vi "Kelvinox_Set_Monitor_Values.vi"(5 "System Monitor Variables (in)":T1) -> (1 "System Monitor Variables (out)":T1)   [LabVIEW 2019]
uses:
  Global/Global Variables/System Monitor Cluster.ctl
  Global/Global Variables/Data_Display_global.vi
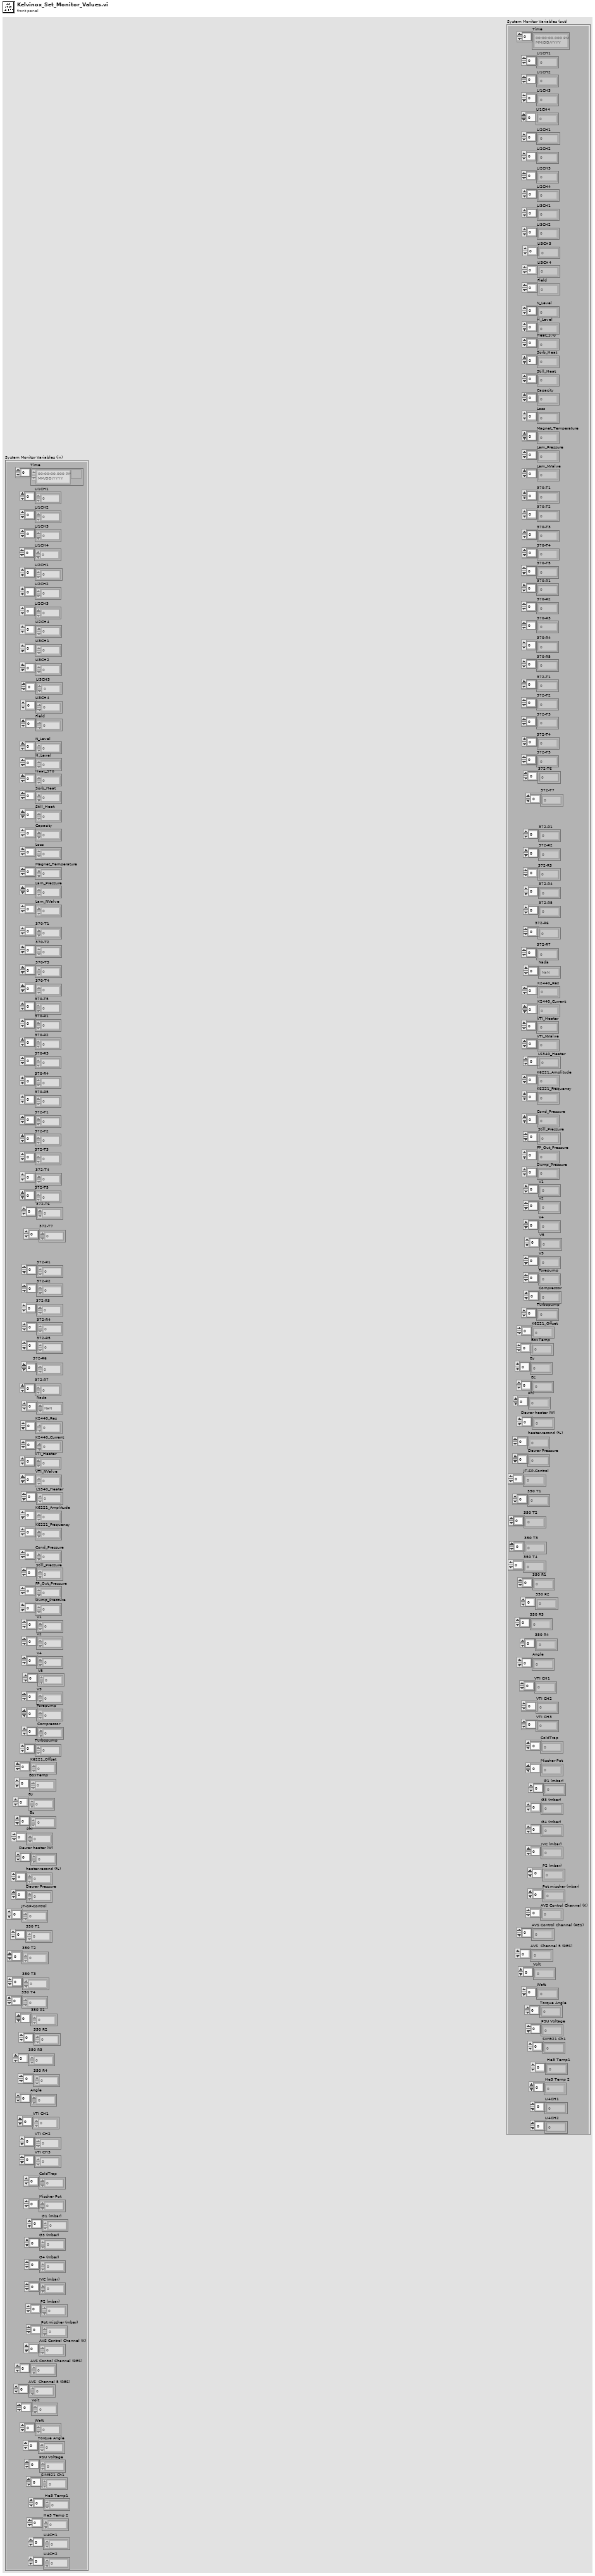
[diagram p1: front panel]
types:
  T1 = typedef "System Monitor Cluster.ctl" = cluster{"Time":timestamp[], "LI1CH1":dbl[], "LI1CH2":dbl[], "LI2CH1":dbl[], "LI2CH2":dbl[], "LI3CH1":dbl[], "LI3CH2":dbl[], "Field":dbl[], "N_Level":dbl[], "H_Level":dbl[], "Heat_370":dbl[], "Sorb_Heat":dbl[], "Still_Heat":dbl[], "Capacity":dbl[], "Loss":dbl[], "Magnet_Temperature":dbl[], "Lam_Pressure":dbl[], "Lam_NValve":dbl[], "370-T1":dbl[], "370-T2":dbl[], "370-T3":dbl[], "370-T4":dbl[], "370-T5":dbl[], "370-R1":dbl[], "370-R2":dbl[], "370-R3":dbl[], "370-R4":dbl[], "370-R5":dbl[], "372-T1":dbl[], "372-T2":dbl[], "372-T3":dbl[], "372-T4":dbl[], "372-T5":dbl[], "372-T6":dbl[], "372-R1":dbl[], "372-R2":dbl[], "372-R3":dbl[], "372-R4":dbl[], "372-R5":dbl[], "372-R6":dbl[], "Nada":dbl[], "K2440_Res":dbl[], "K2440_Current":dbl[], "VTI_Heater":dbl[], "VTI_NValve":dbl[], "LS340_Heater":dbl[], "K6221_Amplitude":dbl[], "K6221_Frequency":dbl[], "Cond_Pressure":dbl[], "Still_Pressure":dbl[], "FP_Out_Pressure":dbl[], "Dump_Pressure":dbl[], "V1":dbl[], "V2":dbl[], "V4":dbl[], "V5":dbl[], "V9":dbl[], "Forepump":dbl[], "Compressor":dbl[], "K6221_Offset":dbl[], "BoxTemp":dbl[], "By":dbl[], "Bz":dbl[], "Phi":dbl[], "heater-recond (%)":dbl[], "Dewar Pressure ":dbl[], "JT-SP-Control":dbl[], "350 T1":dbl[], "350 T2":dbl[], "350 T3":dbl[], "350 T4":dbl[], "350 R1":dbl[], "350 R2":dbl[], "350 R3":dbl[], "350 R4":dbl[], "Angle":dbl[], "VTI CH1":dbl[], "VTI CH2":dbl[], "VTI CH3":dbl[], "ColdTrap":dbl[], "Mischer Pot":dbl[], "G1 (mbar)":dbl[], "G3 (mbar) ":dbl[], "G4 (mbar)":dbl[], "IVC (mbar)":dbl[], "P2 (mbar) ":dbl[], "Pot mischer (mbar)":dbl[], "AVS Control Channel (K)":dbl[], "AVS Control Channel (RES)":dbl[], "AVS  Channel 5 (RES) ":dbl[], "LI3CH3":dbl[], "LI3CH4":dbl[], "LI1CH3":dbl[], "LI1CH4":dbl[], "LI2CH3":dbl[], "LI2CH4":dbl[], "Volt":dbl[], "Watt":dbl[], "Torque Angle":dbl[], "Dewar heater (W)":dbl[], "PSU Voltage":dbl[], "Turbopump":dbl[], "372-R7":dbl[], "372-T7":dbl[], "SIM921 Ch1":dbl[], " He3 Temp1":dbl[], " He3 Temp 2":dbl[], "LI4CH1":dbl[], "LI4CH2":dbl[]}
  T2 = typedef "Kelvinox_Status.ctl" = cluster{"V1":bool, "V2":bool, "Dump":u16, "V4":bool, "V5":bool, "V9":bool, "P1":dbl, "P2":dbl, "P3":dbl, "P4":dbl, "P5":dbl, "Turbo":bool, "Forepump":bool, "speed":dbl, "Sorb":dbl, "1K Pot":dbl, "Still":dbl, "Cold\nPlate":dbl, "MC":dbl, "4K":dbl, "Sample":dbl, "T-Setpoint":dbl, "MC Heater":dbl, "Still Heater":dbl, "Sorb Heater":dbl, "T Control active":bool, "Sorb Res":dbl, "1K Pot Res":dbl, "Still Res":dbl, "Cold Plate Res":dbl, "MC Res":dbl, "4K Res":dbl, "Sample Res":dbl, "Ramping":bool}
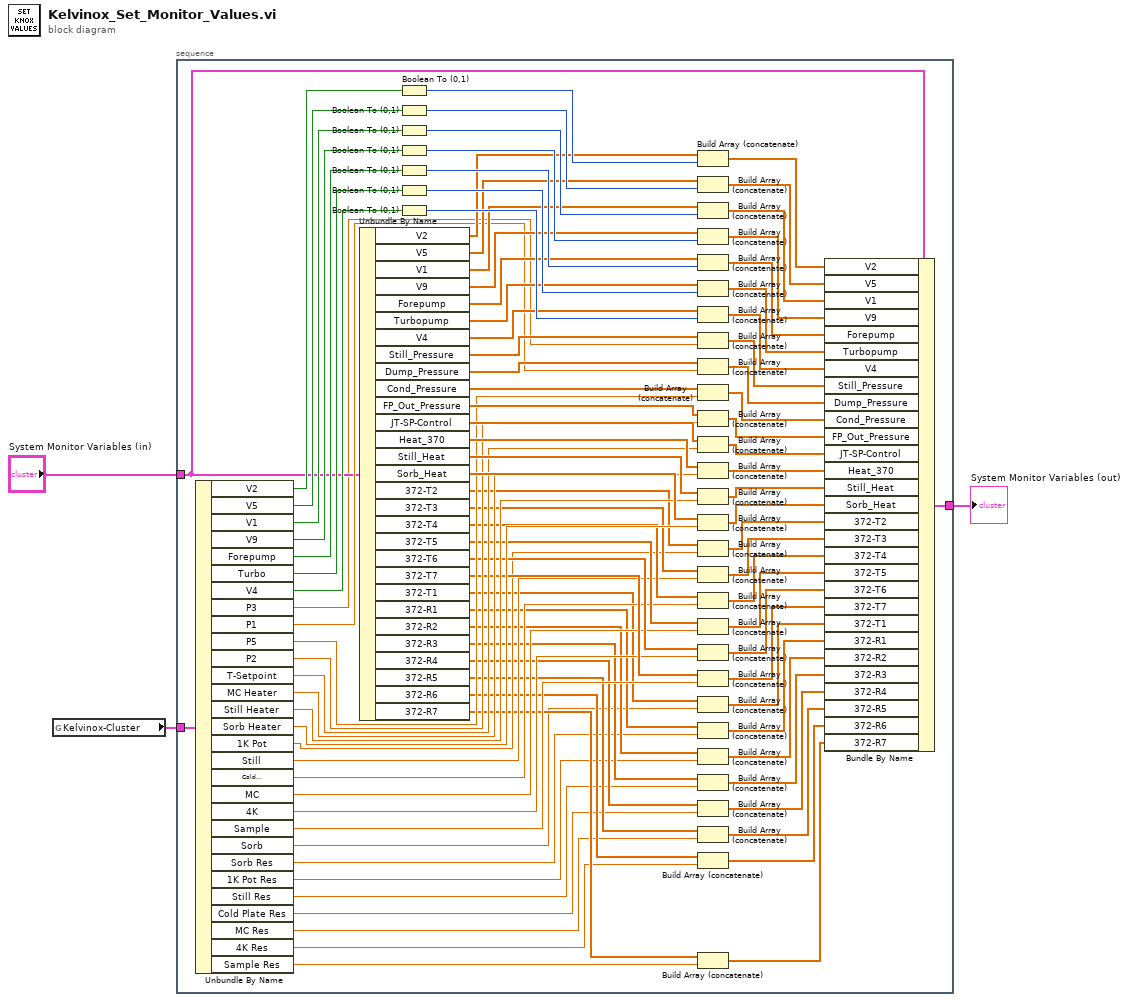
[diagram p0: block diagram]
diagram:
  n1 = global read "Data_Display_global.vi" "Kelvinox-Cluster"() -> (w1:T2)
  n2 = stacked-sequence {
    tunnel: "System Monitor Variables (in)" -> [w51]
    tunnel: [w62] -> w2
    tunnel: w1 -> [w100]
    frame #0 {
      n3 = Unbundle By Name(w100) -> ("V2"=w61:bool, "V5"=w60:bool, "V1"=w59:bool, "V9"=w58:bool, "Forepump"=w57:bool, "Turbo"=w56:bool, "V4"=w55:bool, "P3"=w50:dbl, "P1"=w52:dbl, "P5"=w54:dbl, "P2"=w53:dbl, "T-Setpoint"=w49:dbl, "MC Heater"=w48:dbl, "Still Heater"=w47:dbl, "Sorb Heater"=w46:dbl, "1K Pot"=w39:dbl, "Still"=w38:dbl, "Cold\nPlate"=w37:dbl, "MC"=w36:dbl, "4K"=w35:dbl, "Sample"=w34:dbl, "Sorb"=w19:dbl, "Sorb Res"=w18:dbl, "1K Pot Res"=w17:dbl, "Still Res"=w16:dbl, "Cold Plate Res"=w9:dbl, "MC Res"=w8:dbl, "4K Res"=w15:dbl, "Sample Res"=w14:dbl)
      n4 = Unbundle By Name(w51) -> ("V2"=w79:dbl[], "V5"=w80:dbl[], "V1"=w78:dbl[], "V9"=w82:dbl[], "Forepump"=w84:dbl[], "Turbopump"=w83:dbl[], "V4"=w85:dbl[], "Still_Pressure"=w86:dbl[], "Dump_Pressure"=w87:dbl[], "Cond_Pressure"=w88:dbl[], "FP_Out_Pressure"=w89:dbl[], "JT-SP-Control"=w90:dbl[], "Heat_370"=w91:dbl[], "Still_Heat"=w92:dbl[], "Sorb_Heat"=w93:dbl[], "372-T2"=w45:dbl[], "372-T3"=w44:dbl[], "372-T4"=w43:dbl[], "372-T5"=w42:dbl[], "372-T6"=w41:dbl[], "372-T7"=w40:dbl[], "372-T1"=w27:dbl[], "372-R1"=w26:dbl[], "372-R2"=w25:dbl[], "372-R3"=w24:dbl[], "372-R4"=w23:dbl[], "372-R5"=w22:dbl[], "372-R6"=w21:dbl[], "372-R7"=w20:dbl[])
      n5 = Boolean To (0,1)(Boolean=w61) -> (0, 1=w99:i16)
      n6 = Boolean To (0,1)(Boolean=w60) -> (0, 1=w98:i16)
      n7 = Boolean To (0,1)(Boolean=w59) -> (0, 1=w81:i16)
      n8 = Boolean To (0,1)(Boolean=w58) -> (0, 1=w97:i16)
      n9 = Boolean To (0,1)(Boolean=w57) -> (0, 1=w96:i16)
      n10 = Boolean To (0,1)(Boolean=w56) -> (0, 1=w95:i16)
      n11 = Boolean To (0,1)(Boolean=w55) -> (0, 1=w94:i16)
      n12 = Build Array (concatenate)(w79, w99) -> (w77:dbl[])
      n13 = Build Array (concatenate)(w80, w98) -> (w76:dbl[])
      n14 = Build Array (concatenate)(w78, w81) -> (w75:dbl[])
      n15 = Build Array (concatenate)(w82, w97) -> (w74:dbl[])
      n16 = Build Array (concatenate)(w84, w96) -> (w73:dbl[])
      n17 = Build Array (concatenate)(w83, w95) -> (w72:dbl[])
      n18 = Build Array (concatenate)(w85, w94) -> (w71:dbl[])
      n19 = Build Array (concatenate)(w86, w50) -> (w70:dbl[])
      n20 = Build Array (concatenate)(w87, w52) -> (w69:dbl[])
      n21 = Build Array (concatenate)(w88, w54) -> (w68:dbl[])
      n22 = Build Array (concatenate)(w89, w53) -> (w67:dbl[])
      n23 = Build Array (concatenate)(w90, w49) -> (w66:dbl[])
      n24 = Build Array (concatenate)(w91, w48) -> (w65:dbl[])
      n25 = Build Array (concatenate)(w92, w47) -> (w64:dbl[])
      n26 = Build Array (concatenate)(w93, w46) -> (w63:dbl[])
      n27 = Build Array (concatenate)(w45, w39) -> (w33:dbl[])
      n28 = Build Array (concatenate)(w44, w38) -> (w32:dbl[])
      n29 = Build Array (concatenate)(w43, w37) -> (w31:dbl[])
      n30 = Build Array (concatenate)(w42, w36) -> (w30:dbl[])
      n31 = Build Array (concatenate)(w41, w35) -> (w29:dbl[])
      n32 = Build Array (concatenate)(w40, w34) -> (w28:dbl[])
      n33 = Build Array (concatenate)(w27, w19) -> (w13:dbl[])
      n34 = Build Array (concatenate)(w26, w18) -> (w12:dbl[])
      n35 = Build Array (concatenate)(w25, w17) -> (w11:dbl[])
      n36 = Build Array (concatenate)(w24, w16) -> (w10:dbl[])
      n37 = Build Array (concatenate)(w23, w9) -> (w7:dbl[])
      n38 = Build Array (concatenate)(w22, w8) -> (w6:dbl[])
      n39 = Build Array (concatenate)(w21, w15) -> (w5:dbl[])
      n40 = Build Array (concatenate)(w20, w14) -> (w4:dbl[])
      n41 = Bundle By Name(cluster=w51, "V2"=w77, "V5"=w76, "V1"=w75, "V9"=w74, "Forepump"=w73, "Turbopump"=w72, "V4"=w71, "Still_Pressure"=w70, "Dump_Pressure"=w69, "Cond_Pressure"=w68, "FP_Out_Pressure"=w67, "JT-SP-Control"=w66, "Heat_370"=w65, "Still_Heat"=w64, "Sorb_Heat"=w63, "372-T2"=w33, "372-T3"=w32, "372-T4"=w31, "372-T5"=w30, "372-T6"=w29, "372-T7"=w28, "372-T1"=w13, "372-R1"=w12, "372-R2"=w11, "372-R3"=w10, "372-R4"=w7, "372-R5"=w6, "372-R6"=w5, "372-R7"=w4) -> (w62:T1)
    }
  }
  "System Monitor Variables (out)" <- w2
